vi "Get PStar Vector.vi"(8 "error in (no error)":errorcluster, 10 "q":dbl, 11 "link in":refnum<class "NI_Robotics_Link.lvclass">) -> (0 "error out":errorcluster, 2 "p*":dbl[](array[numeric]), 3 "link out":refnum<class "NI_Robotics_Link.lvclass">)   [LabVIEW 2017, in "NI_Robotics_Link.lvclass"]
uses:
  <vilib>/robotics/Kinematics/Link/NI_Robotics_Link.lvclass
  <vilib>/robotics/Kinematics/Link/NI_Robotics_Link.lvclass/NI_Robotics_Link.ctl
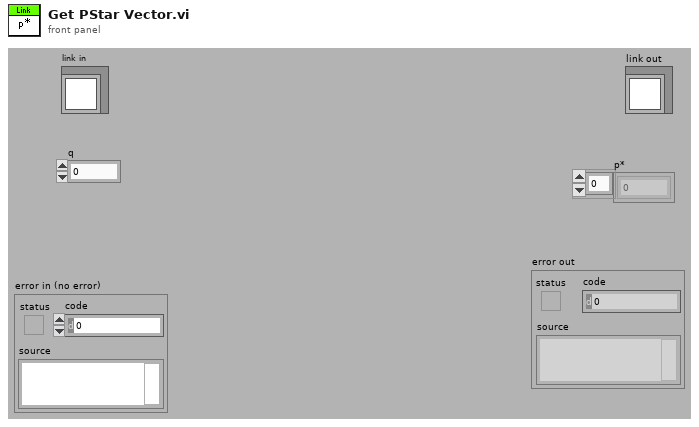
[diagram p1: front panel]
types:
  T1 = typedef "NI_Robotics_Link.lvclass/Joint Type.ctl" = enum16{"Revolute", "Prismatic"}
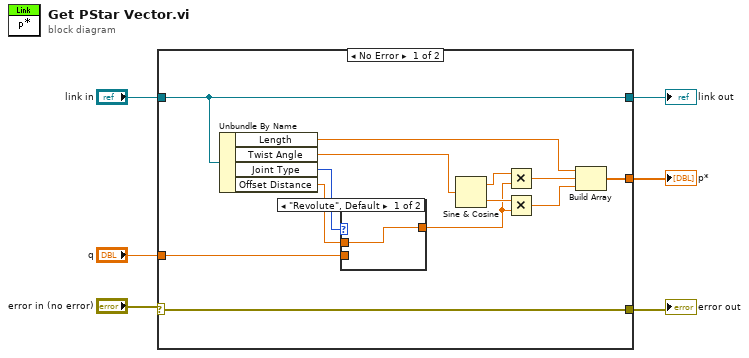
[diagram p0: block diagram]
diagram:
  n1 = case shown="No Error" "error in (no error)" {
    selector: "error in (no error)" -> [w8 w23]
    tunnel: "link in" -> [w7 w22]
    tunnel: [w19 _] -> w5
    tunnel: "q" -> [w16 _]
    tunnel: [w8 w23] -> w2
    tunnel: [w7 w22] -> w1
    frame No Error {
      n2 = Unbundle By Name(w7) -> ("Length"=w10:dbl, "Twist Angle"=w9:dbl, "Joint Type"=w15:T1, "Offset Distance"=w14:dbl)
      n3 = case shown="\"Revolute\", Default" w15 {
        tunnel: w16 -> [_ w21]
        tunnel: [w20 w21] -> w13
        tunnel: w14 -> [w20 _]
        frame "Revolute", Default {
        }
        frame "Prismatic" {
        }
      }
      n4 = Sine & Cosine(0:w9) -> (1:w18:dbl, 2:w17:dbl)
      n5 = Multiply(x=w18, y=w13) -> (x*y=w12:dbl)
      n6 = Multiply(x=w17, y=w13) -> (x*y=w11:dbl)
      n7 = Build Array(w10, w12, w11) -> (w19:dbl[])
    }
    frame Error {
    }
  }
  "link out" <- w1
  "p*" <- w5
  "error out" <- w2
